vi "brokenvi - dependent VI in lower LV.vi"   [LabVIEW 2021]
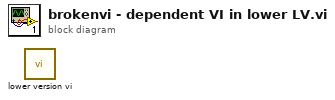
[diagram p0: block diagram]
diagram:
  n1 = call "lower version vi.vi"() -> ()  [unwired: 11 in, 1 out]
